vi "MoveScanTask.vi"(6 "Multi ScanPar":bool[](array[boolean]), 7 "ActScanPar":bool[](array[boolean]), 8 "ErrorIn(No Error)":errorcluster caption="entrée d'erreur (pas d'erreur)", 9 "ScanFuncArrIn":string[][](array[string]), 10 "Dir(Up:T)":bool, 11 "TaskIdx":i32) -> (0 "sortie d'erreur":errorcluster, 1 "ScanFuncArrOut":string[][](array[string]), 2 "ScanFuncOut":string, 4 "Multi ScanParOut":bool[](array[boolean]), 5 "ActScanParOut":bool[](array[boolean]))   [LabVIEW 2019]
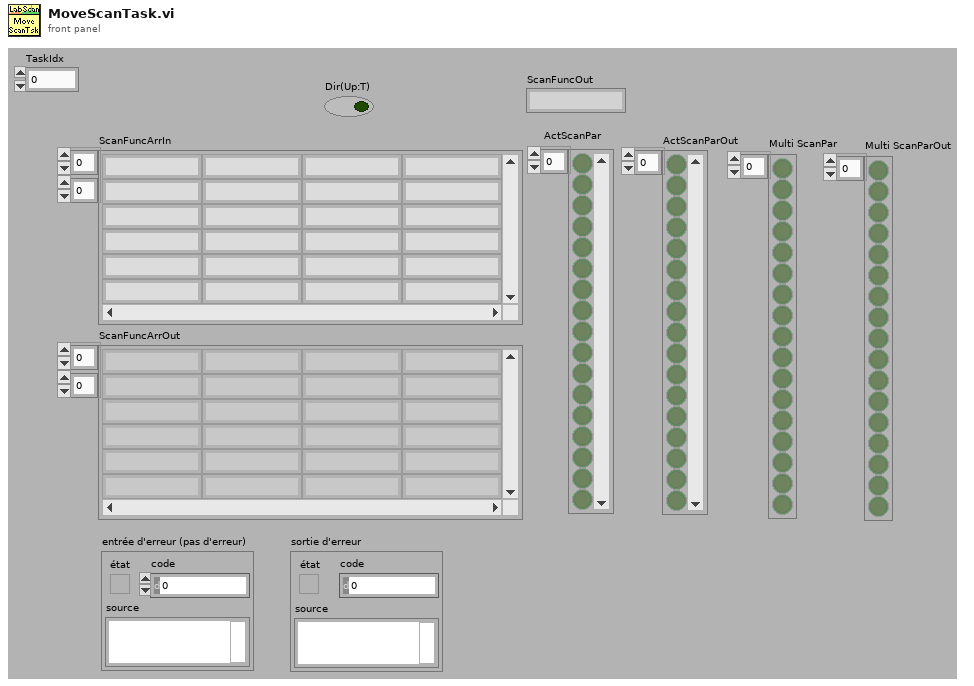
[diagram p1: front panel]
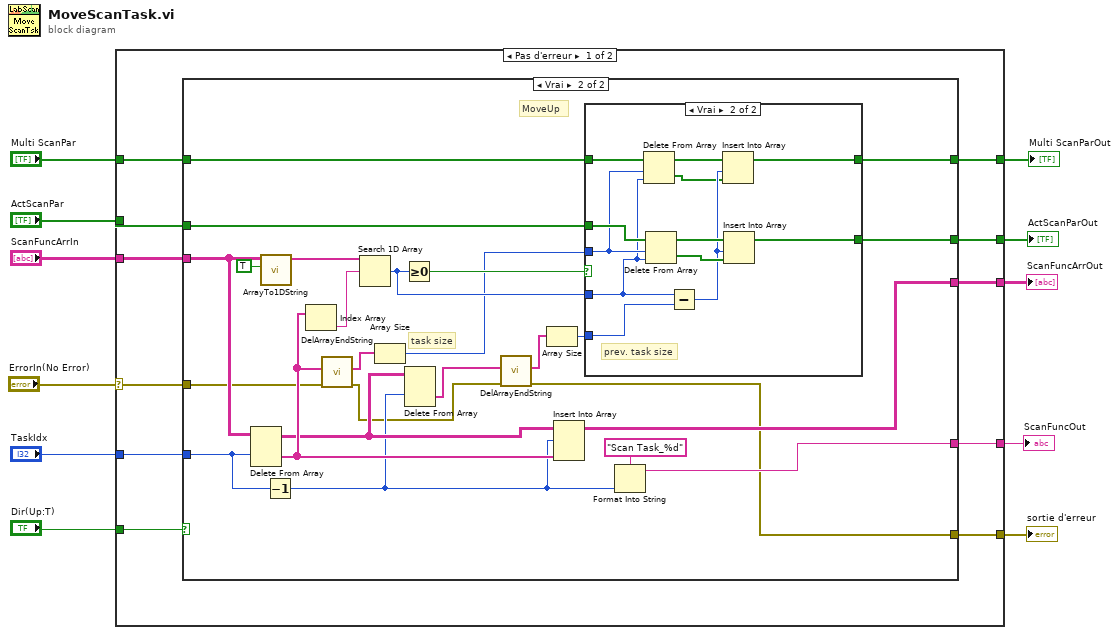
[diagram p0: block diagram]
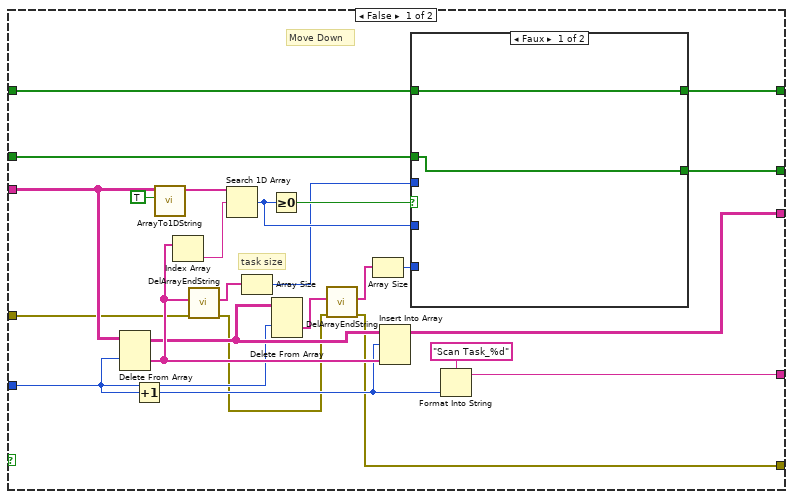
[diagram p2: hidden frame]
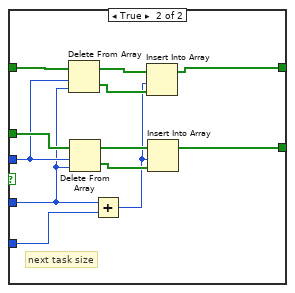
[diagram p3: hidden frame]
diagram:
  n1 = case shown="Pas d'erreur" "ErrorIn(No Error)" {
    selector: "ErrorIn(No Error)" -> [w15 w104]
    tunnel: "ScanFuncArrIn" -> [w22 w103]
    tunnel: "Dir(Up:T)" -> [w20 _]
    tunnel: [w16 w104] -> w8
    tunnel: [w18 w103] -> w7
    tunnel: "ActScanPar" -> [w17 w102]
    tunnel: [w14 w102] -> w5
    tunnel: "TaskIdx" -> [w21 _]
    tunnel: [w19 _] -> w3
    tunnel: [w13 w101] -> w2
    tunnel: "Multi ScanPar" -> [w12 w101]
    frame No Error {
      n2 = case shown="Vrai" w20 {
        tunnel: w22 -> [w44 w83]
        tunnel: w21 -> [w27 w82]
        tunnel: [w43 w81] -> w19
        tunnel: [w42 w80] -> w18
        tunnel: w17 -> [w39 w77]
        tunnel: [w25 w64] -> w16
        tunnel: w15 -> [w34 w72]
        tunnel: [w28 w66] -> w14
        tunnel: [w23 w63] -> w13
        tunnel: w12 -> [w24 w62]
        frame False {
          # "Move Down"
          # "task size"
          n3 = Delete From Array(array=w44, index (row)=w27) -> (deleted portion=w36:string[], array with subset deleted=w33:string[][])  [unwired: 2 in]
          n4 = Increment(x=w27) -> (x+1=w32:i32)
          n5 = call <userlib>:"ArrayTo1DString.vi"("DelArrEnd(F)"=TRUE ("DelArrEnd"), "tableau"=w44) -> ("Array Out"=w47:string[])  [unwired: 7 in, 2 out]
          n6 = Index Array(array=w36) -> (element=w41:string)  [unwired: 1 in]
          n7 = call <userlib>:"DelArrayEndString.vi"("ErrorIn(No Error)"=w34, "Array In"=w36) -> ("sortie d'erreur"=w26:errorcluster, "Array Out"=w35:string[])  [unwired: 8 in]
          n8 = Search 1D Array(1D array=w47, element=w41) -> (index of element=w38:i32)  [unwired: 1 in]
          n9 = Array Size(array=w35) -> (size(s)=w37:i32)
          n10 = Greater Or Equal To 0?(x=w38) -> (x >= 0?=w40:bool)
          n11 = Delete From Array(array=w33, index (row)=w27) -> (deleted portion=w30:string[])  [unwired: 2 in, 1 out]
          n12 = call <userlib>:"DelArrayEndString.vi"("ErrorIn(No Error)"=w26, "Array In"=w30) -> ("sortie d'erreur"=w25:errorcluster, "Array Out"=w31:string[])  [unwired: 8 in]
          n13 = Array Size(array=w31) -> (size(s)=w29:i32)
          n14 = Insert Into Array(array=w33, index (row)=w32, new element=w36) -> (w42:string[][])  [unwired: 1 in]
          n15 = case shown="Faux" w40 {
            tunnel: w39 -> [w49 w61]
            tunnel: w38 -> [_ w50]
            tunnel: w37 -> [_ w51]
            tunnel: w29 -> [_ w60]
            tunnel: [w49 w57] -> w28
            tunnel: w24 -> [w48 w54]
            tunnel: [w48 w53] -> w23
            frame False {
            }
            frame True {
              # "next task size"
              n16 = Delete From Array(array=w54, length=w51, index=w50) -> (deleted portion=w55:bool[], array with subset deleted=w56:bool[])
              n17 = Delete From Array(array=w61, length=w51, index=w50) -> (deleted portion=w58:bool[], array with subset deleted=w59:bool[])
              n18 = Add(x=w50, y=w60) -> (x+y=w52:i32)
              n19 = Insert Into Array(array=w56, index=w52, new element=w55) -> (w53:bool[])
              n20 = Insert Into Array(array=w59, index=w52, new element=w58) -> (w57:bool[])
            }
          }
          n21 = Format Into String(format string="Scan Task_%d" ("chaîne de format"), w32) -> (resulting string=w43:string)  [unwired: 2 in, 1 out]
        }
        frame True {
          # "MoveUp"
          # "task size"
          n22 = Delete From Array(array=w83, index (row)=w82) -> (deleted portion=w74:string[], array with subset deleted=w71:string[][])  [unwired: 2 in]
          n23 = call <userlib>:"ArrayTo1DString.vi"("DelArrEnd(F)"=TRUE ("DelArrEnd"), "tableau"=w83) -> ("Array Out"=w86:string[])  [unwired: 7 in, 2 out]
          n24 = Decrement(x=w82) -> (x-1=w70:i32)
          n25 = Index Array(array=w74) -> (element=w79:string)  [unwired: 1 in]
          n26 = call <userlib>:"DelArrayEndString.vi"("ErrorIn(No Error)"=w72, "Array In"=w74) -> ("sortie d'erreur"=w65:errorcluster, "Array Out"=w73:string[])  [unwired: 8 in]
          n27 = Search 1D Array(1D array=w86, element=w79) -> (index of element=w76:i32)  [unwired: 1 in]
          n28 = Array Size(array=w73) -> (size(s)=w75:i32)
          n29 = Greater Or Equal To 0?(x=w76) -> (x >= 0?=w78:bool)
          n30 = Delete From Array(array=w71, index (row)=w70) -> (deleted portion=w68:string[])  [unwired: 2 in, 1 out]
          n31 = call <userlib>:"DelArrayEndString.vi"("ErrorIn(No Error)"=w65, "Array In"=w68) -> ("sortie d'erreur"=w64:errorcluster, "Array Out"=w69:string[])  [unwired: 8 in]
          n32 = Array Size(array=w69) -> (size(s)=w67:i32)
          n33 = Insert Into Array(array=w71, index (row)=w70, new element=w74) -> (w80:string[][])  [unwired: 1 in]
          n34 = case shown="Vrai" w78 {
            tunnel: w77 -> [w88 w100]
            tunnel: w76 -> [_ w91]
            tunnel: w75 -> [_ w92]
            tunnel: w67 -> [_ w99]
            tunnel: [w88 w96] -> w66
            tunnel: [w87 w94] -> w63
            tunnel: w62 -> [w87 w93]
            frame False {
            }
            frame True {
              # "prev. task size"
              n35 = Delete From Array(array=w93, length=w92, index=w91) -> (deleted portion=w90:bool[], array with subset deleted=w89:bool[])
              n36 = Delete From Array(array=w100, length=w92, index=w91) -> (deleted portion=w97:bool[], array with subset deleted=w98:bool[])
              n37 = Subtract(x=w91, y=w99) -> (x-y=w95:i32)
              n38 = Insert Into Array(array=w89, index=w95, new element=w90) -> (w94:bool[])
              n39 = Insert Into Array(array=w98, index=w95, new element=w97) -> (w96:bool[])
            }
          }
          n40 = Format Into String(format string="Scan Task_%d" ("chaîne de format"), w70) -> (resulting string=w81:string)  [unwired: 2 in, 1 out]
        }
      }
    }
    frame Error {
    }
  }
  "sortie d'erreur" <- w8
  "ScanFuncArrOut" <- w7
  "ActScanParOut" <- w5
  "ScanFuncOut" <- w3
  "Multi ScanParOut" <- w2
